vi "Set Batch Name.vi"(0 "VISA resource name":refnum<visa-resource-name>, 5 "Batch Number (\"\")":string, 7 "Lot Number (0)":i32, 11 "error in (no error)":errorcluster) -> (4 "VISA resource name out":refnum<visa-resource-name>, 15 "error out":errorcluster)   [LabVIEW 2020, in "Yokogawa GX Series.lvlib"]
doc: "Sets the batch name.\n\nCommand: OBatName"
uses:
  <instrlib>/Yokogawa GX Series/Yokogawa GX Series.lvlib
panel:
  in  "Batch Group Number  (0: OFF)":i32(ring) items=["OFF", "1", "2", "3", "4", "5", "6", "7", "8", "9", "10", "11", "12"]
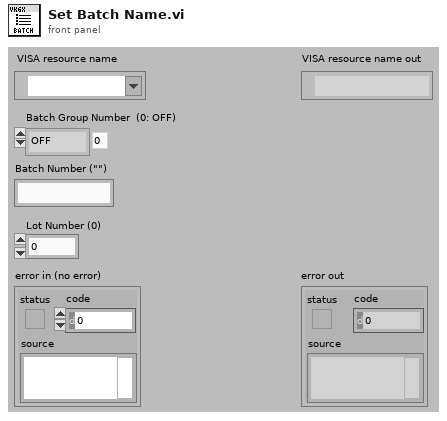
[diagram p1: front panel]
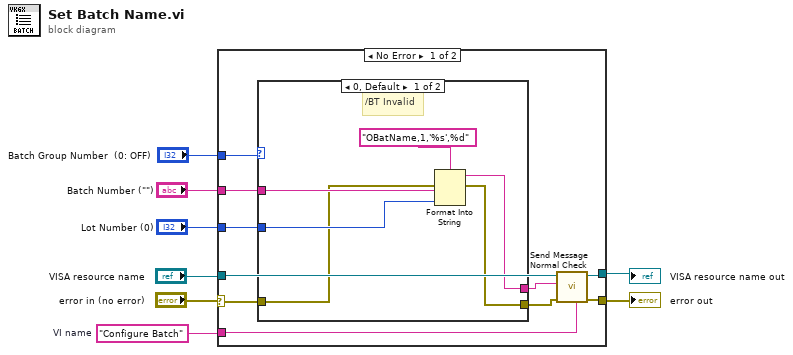
[diagram p0: block diagram]
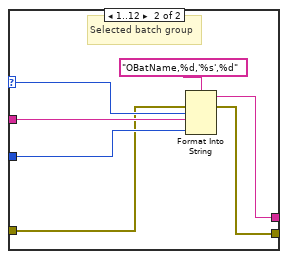
[diagram p2: hidden frame]
diagram:
  w7 = "Configure Batch"  # VI name
  n1 = case shown="No Error" "error in (no error)" {
    selector: "error in (no error)" -> [w9 w32]
    tunnel: "VISA resource name" -> [w18 w33]
    tunnel: w7 -> [w17 _]
    tunnel: [w16 w33] -> w6
    tunnel: [w15 w32] -> w5
    tunnel: "Batch Number (\"\")" -> [w13 _]
    tunnel: "Lot Number (0)" -> [w12 _]
    tunnel: "Batch Group Number  (0: OFF)" -> [w14 _]
    frame No Error {
      n2 = case shown="0, Default" w14 {
        selector: w14 -> [_ w29]
        tunnel: [w24 w31] -> w10
        tunnel: [w23 w30] -> w11
        tunnel: w13 -> [w21 w27]
        tunnel: w12 -> [w20 w26]
        tunnel: w9 -> [w19 w25]
        frame 0, Default {
          # "/BT Invalid"
          n3 = Format Into String(format string="OBatName,1,'%s',%d", error in=w19, w21, w20) -> (resulting string=w23:string, error out=w24:errorcluster)  [unwired: 1 in]
        }
        frame 1..12 {
          # "Selected batch group"
          n4 = Format Into String(format string="OBatName,%d,'%s',%d", error in=w25, w29, w27, w26) -> (resulting string=w30:string, error out=w31:errorcluster)  [unwired: 1 in]
        }
      }
      n5 = call <instrlib>:"Send Message Normal Check.vi"("Source (\"\")"=w17, "error in (no error)"=w10, "Send Message (\"\")"=w11, "VISA resource name"=w18) -> ("error out"=w15:errorcluster, "VISA resource name out"=w16:refnum<visa-resource-name>)  [unwired: 2 in, 4 out]
    }
    frame Error {
    }
  }
  "error out" <- w5
  "VISA resource name out" <- w6
